vi "Copy Memory Address to Image.vi"   [LabVIEW 2020, in "image.lvlib"]
doc: "Copy the Memory Source Data into the Destinaton Image.\n\nThe destination image will be resized to accomodate the memory source data.\n\n<b>Ensure the Source Parameters are correct to avoid memory corruption.</b>"
uses:
  image.lvlib
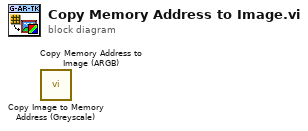
[diagram p0: block diagram]
diagram:
  n1 = call "Copy Image to Memory Address (Greyscale).vi"() -> ()  [unwired: 10 in, 2 out]
  n2 = call "Copy Memory Address to Image (ARGB).vi"() -> ()  [unwired: 10 in, 2 out]
